vi "Clear Busy.vi"(8 "error in (no error)":errorcluster, 11 "Process State":refnum<data-value>) -> (0 "error out":errorcluster, 3 "Process State":refnum<data-value>)   [LabVIEW 2022 SP3, in "Process State Data.lvclass"]
uses:
  Process State Data.lvclass
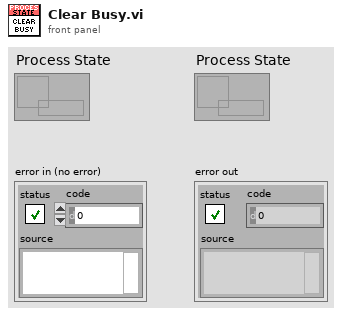
[diagram p1: front panel]
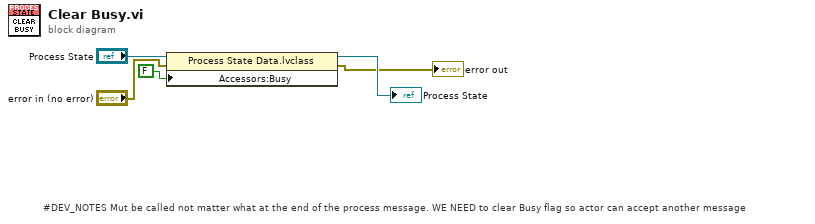
[diagram p0: block diagram]
diagram:
  # "#DEV_NOTES Mut be called not matter what at the end of the process message. WE NEED to clear Busy flag so actor can accept another message"
  n1 = property class="Process State Data.lvclass"(reference="Process State", error in="error in (no error)", "Accessors:Busy"=FALSE ("Busy")) -> (reference out=→"Process State":refnum<data-value>, error out=→"error out":errorcluster)
